vi "Untitled 2.vi"() -> ()   [LabVIEW 2014]
uses:
  <vilib>/Utility/file.llb/Write To Spreadsheet File (I64).vi
panel:
  in  "Path":path
  in  "stop (F) 2":bool caption="stop (F)"
  out "Waveform Graph":dynamicdata(graph)
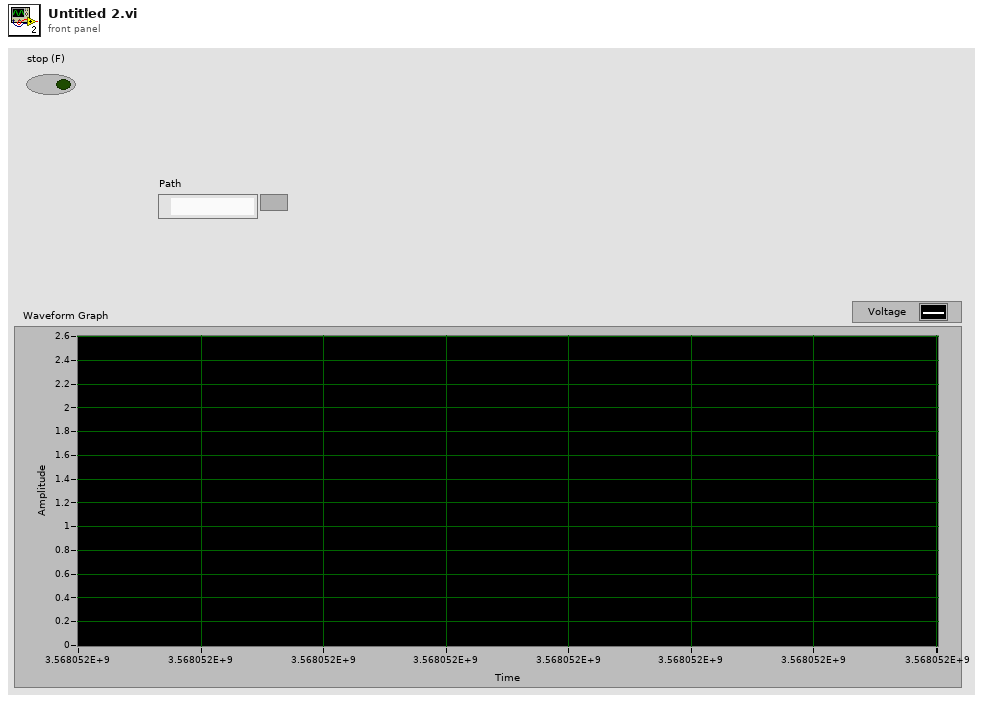
[diagram p1: front panel]
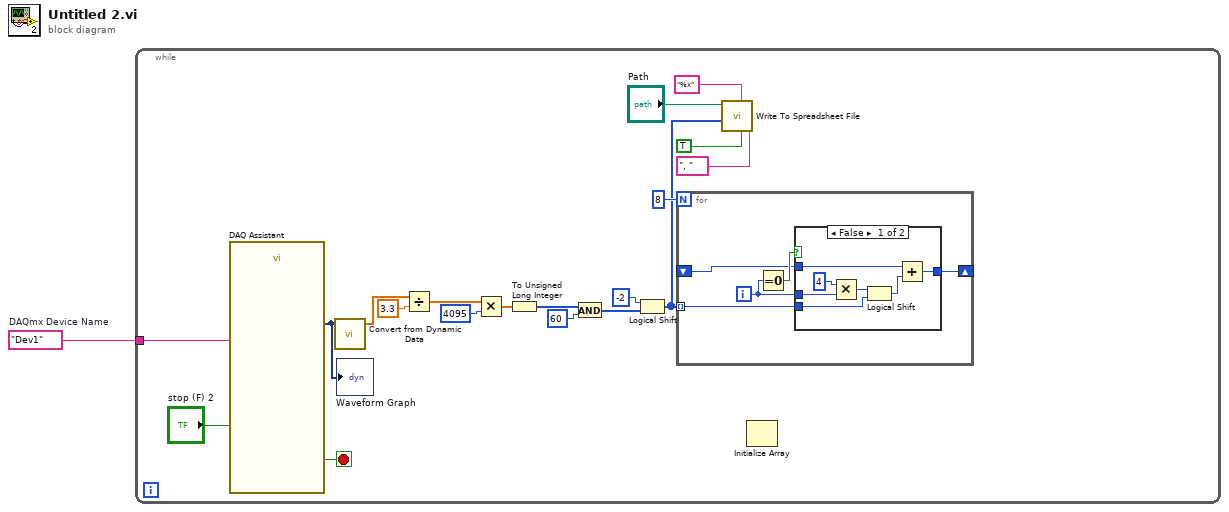
[diagram p0: block diagram]
diagram:
  w1 = tag "Dev1"  # DAQmx Device Name
  n1 = while {
    tunnel: w1 -> [w18]
    stop <- w20 stop-if-true
    n2 = call "DAQ Assistant"("stop (F)"="stop (F) 2", "device name"=w18) -> ("data"=w7:dynamicdata, "stopped"=w20:bool)  [unwired: 14 in, 2 out]
    "Waveform Graph" <- w7
    n3 = call "Convert from Dynamic Data"("Dynamic Data Type"=w7) -> ("Array"=w8:dbl[])  [unwired: 3 in]
    n4 = Divide(x=w8, y=3.3) -> (x/y=w16:dbl[])
    n5 = Multiply(x=w16, y=4095) -> (x*y=w14:dbl[])
    n6 = To Unsigned Long Integer(number=w14) -> (unsigned 32bit integer=w13:u32[])
    n7 = And(x=w13, y=u32 60) -> (x .and. y?=w11:u32[])
    n8 = Logical Shift(y=-2, x=w11) -> (x << y=w2:u32[])
    n9 = for {
      N: 8 -> [_]
      tunnel: w2 -> [w24] mode=indexing
      shift-right: [w22] -> _
      shift-left: _ -> [w21]
      i -> [w23]
      n10 = Equal To 0?(x=w23) -> (x = 0?=w25:bool)
      n11 = case shown="False" w25 {
        tunnel: w24 -> [w30 w33]
        tunnel: w23 -> [w32 _]
        tunnel: [w26 w33] -> w22
        tunnel: w21 -> [w28 _]
        frame False {
          n12 = Multiply(x=4, y=w32) -> (x*y=w29:i32)
          n13 = Logical Shift(y=w29, x=w30) -> (x << y=w27:u32)
          n14 = Add(x=w28, y=w27) -> (x+y=w26:u32)
        }
        frame True {
        }
      }
    }
    n15 = call-poly <vilib>:"Write To Spreadsheet File.vi"("delimiter (\\t)"=", ", "transpose? (no:F)"=TRUE, "format (%d)"="%x", "1D data"=w2, "file path (dialog if empty)"="Path") -> ()  [unwired: 3 in, 1 out]
    n16 = Initialize Array() -> ()  [unwired: 2 in, 1 out]
  }
